vi "GFGsaveAllToFile.vi"(8 "error in":errorcluster, 11 "file path":path) -> (0 "error out":errorcluster)   [LabVIEW 2012, in "GFG library.lvlib"]
uses:
  GFGallGet.vi
  GFG library.lvlib
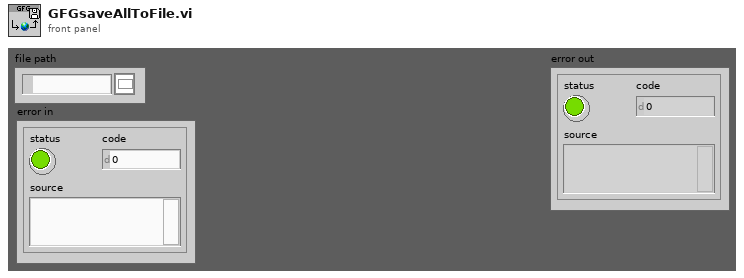
[diagram p1: front panel]
types:
  T1 = enum16{"open", "replace", "create", "open or create", "replace or create", "replace or create with confirmation"}
  T2 = typedef "VariantType.lvlib/Type.ctl" = enum8{"Invalid Type", "Void", "I8", "I16", "I32", "I64", "U8", "U16", "U32", "U64", "Single Float", "Double Float", "Extended Float", "Single Complex", "Double Complex", "Extended Complex", "Enum U8", "Enum U16", "Enum U32", "Enum U64", "Single Float With Unit", "Double Float With Unit", "Extended Float With Unit", "Single Complex with Unit", "Double Complex with Unit", "Extended Complex with Unit", "Boolean", "String", "Path", "Picture", "Tag", "Array", "Cluster", "Variant", "LV Variant", "Waveform", "Timestamp", "Digital Waveform", "Digital Data", "ExpressData", "Refnum", "External Data", "VI", "Poly VI", "LabVIEW Class Instance", "Fixed Point"}
  T3 = cluster{"Variable Name Out":string, "Data Type Out":T2, "Variant Out":variant}[]
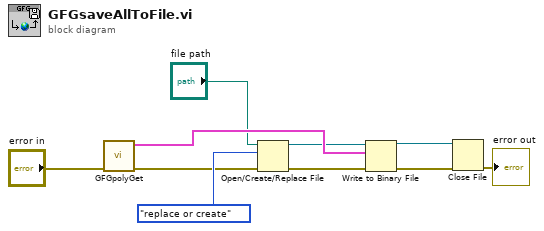
[diagram p0: block diagram]
diagram:
  n1 = call-poly "GFGpolyGet.vi"("error in (no error)"="error in") -> ("error out"=w4:errorcluster, "Array of Clusters of Variables"=w10:T3)  [unwired: 9 in]
  n2 = Open/Create/Replace File(file path (use dialog)="file path", error in=w4, operation (0:open)=T1."replace or create") -> (refnum out=w8:refnum<file>, error out=w6:errorcluster)  [unwired: 3 in, 1 out]
  n3 = Write to Binary File(file (use dialog)=w8, data=w10, error in=w6) -> (refnum out=w2:refnum<file>, error out=w3:errorcluster)  [unwired: 3 in, 1 out]
  n4 = Close File(refnum=w2, error in=w3) -> (error out=→"error out":errorcluster)  [unwired: 1 out]
